vi "单通道闪烁&颜色.vi"(4 "灭阈值":i32=100, 5 "读取时间s":dbl=1.5, 6 "亮阈值":i32=300, 7 "地址":string="02", 8 "error in (no error)":errorcluster caption="错误输入（无错误）", 9 "颜色选择":enum16{"红", "绿", "蓝", "白", "黄", "琥珀色"}(ring)=enum."黄", 10 "分析仪通道":T1(ring), 11 "Index":u8) -> (0 "error out":errorcluster caption="错误输出", 1 "结果？":bool, 2 "闪烁？":bool, 3 "颜色？":bool)   [LabVIEW 2015]
panel:
  out "R":u16
  out "G":u16
  out "B":u16
  out "i":u16
  out "循环数据":u16[][](array[numeric])
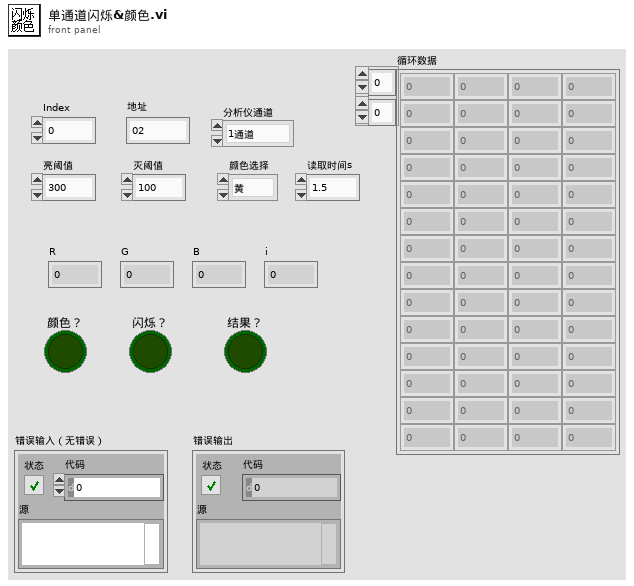
[diagram p1: front panel]
types:
  T1 = enum16{"1通道", "2通道", "3通道", "4通道", "5通道", "6通道", "7通道", "8通道", "9通道", "10通道", "11通道", "12通道", "13通道", "14通道", "15通道", "16通道"}
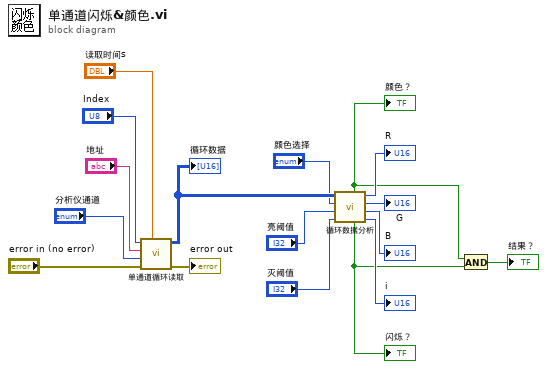
[diagram p0: block diagram]
diagram:
  n1 = call "单通道循环读取.vi"("超时s"="读取时间s", "error in (no error)"="error in (no error)", "分析仪通道"="分析仪通道", "地址"="地址", "MyIndex"="Index") -> ("error out"=→"error out":errorcluster, "循环数据"=w12:u16[][])  [unwired: 4 in, 1 out]
  "循环数据" <- w12
  n2 = call "循环数据分析.vi"("灭阈值"="灭阈值", "亮阈值"="亮阈值", "颜色选择"="颜色选择", "循环数据"=w12) -> ("i"=→"i":u16, "B"=→"B":u16, "G"=→"G":u16, "R"=→"R":u16, "闪烁？"=w3:bool, "颜色结果"=w4:bool)  [unwired: 2 in]
  "闪烁？" <- w3
  "颜色？" <- w4
  n3 = And(x=w4, y=w3) -> (x .and. y?=→"结果？":bool)
